vi "OLA Compute Polarization.vi"(9 "ignore fraction":dbl=0.1875, 10 "cal":dbl=1.0, 11 "signal":dbl[](array[numeric])) -> (2 "polarization":dbl, 3 "area":dbl)   [LabVIEW 2010]
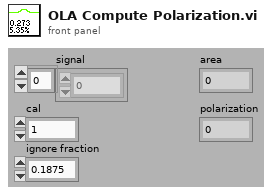
[diagram p1: front panel]
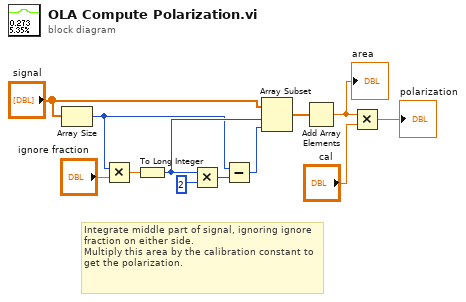
[diagram p0: block diagram]
diagram:
  # "Integrate middle part of signal, ignoring ignore fraction on either side.\nMultiply this area by the calibration constant to get the polarization."
  n1 = Array Size(array="signal") -> (size(s)=w3:i32)
  n2 = Multiply(x=w3, y="ignore fraction") -> (x*y=w10:dbl)
  n3 = To Long Integer(number=w10) -> (32bit integer=w7:i32)
  n4 = Multiply(x=w7, y=2) -> (x*y=w8:i32)
  n5 = Subtract(x=w3, y=w8) -> (x-y=w11:i32)
  n6 = Array Subset(array="signal", index=w7, length=w11) -> (w12:dbl[])
  n7 = Add Array Elements(numeric array=w12) -> (sum=w2:dbl)
  "area" <- w2
  n8 = Multiply(x=w2, y="cal") -> (x*y=→"polarization":dbl)
